vi "Sub01_Pixmap.vi"(8 "error in (no error)":errorcluster, 11 "Image Path":path) -> (0 "error out":errorcluster, 2 "Array":u32[](array[numeric]), 3 "Image Disp":picture)   [LabVIEW 2019]
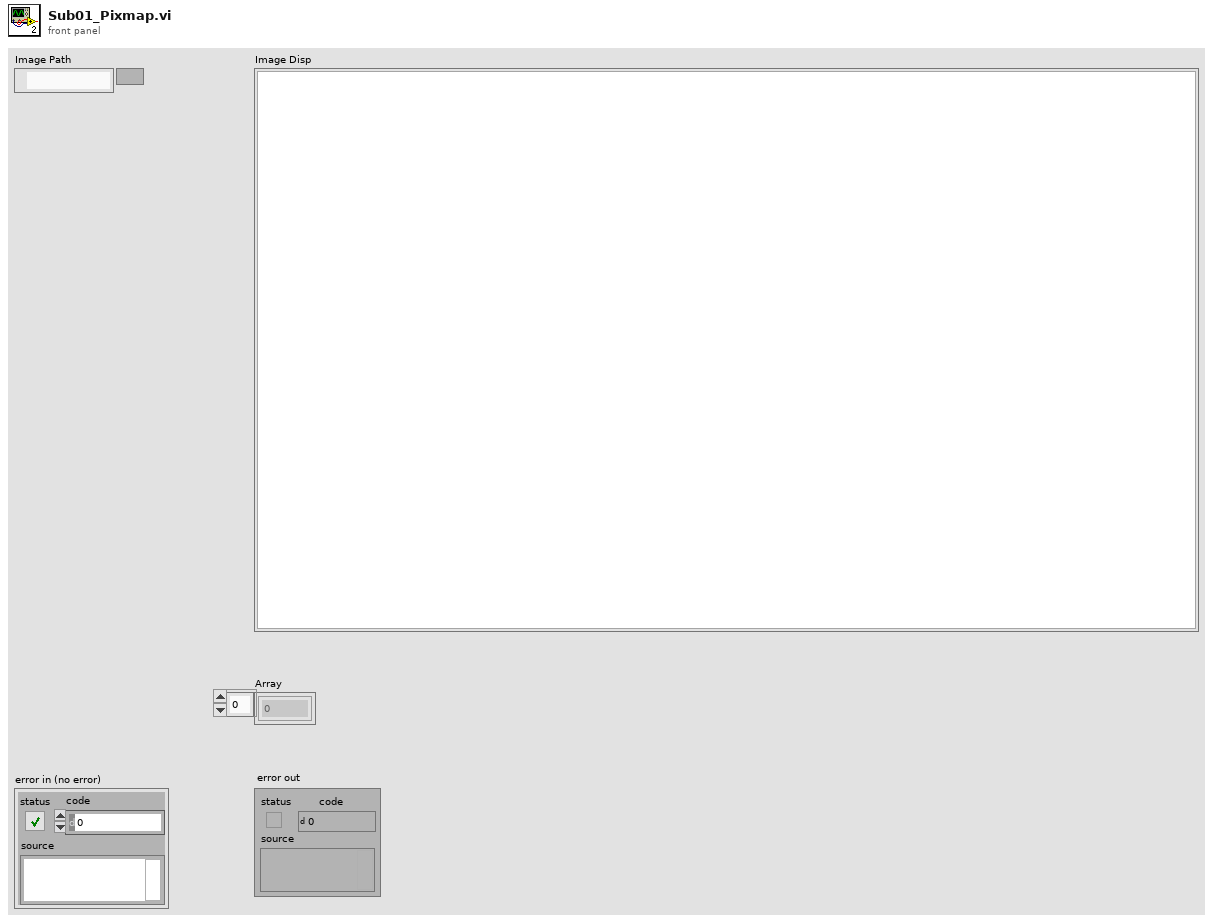
[diagram p1: front panel]
types:
  T1 = typedef "imagedata.ctl" = cluster{"image type":i32, "image depth":i32, "image":u8[], "mask":u8[], "colors":u32[], "Rectangle":cluster{"left":i16, "top":i16, "right":i16, "bottom":i16}}
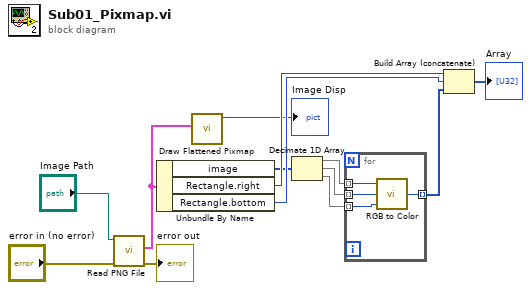
[diagram p0: block diagram]
diagram:
  n1 = call <vilib>:"Read PNG File.vi"("error in (no error)"="error in (no error)", "path to PNG file"="Image Path") -> ("error out"=→"error out":errorcluster, "image data"=w10:T1)  [unwired: 7 in, 1 out]
  n2 = Unbundle By Name(w10) -> ("image"=w5:u8[], "Rectangle.right"=w12:i16, "Rectangle.bottom"=w13:i16)
  n3 = call <vilib>:"Draw Flattened Pixmap.vi"("image data"=w10) -> ("new picture"=→"Image Disp":picture)  [unwired: 8 in]
  n4 = Decimate 1D Array(w5) -> (w4:u8[], w3:u8[], w2:u8[])
  n5 = for {
    tunnel: w4 -> [w17] mode=indexing
    tunnel: w3 -> [w16] mode=indexing
    tunnel: w2 -> [w14] mode=indexing
    tunnel: [w15] -> w1 mode=indexing
    n6 = call <vilib>:"RGB to Color.vi"("B"=w14, "G"=w16, "R"=w17) -> ("Color"=w15:u32)
  }
  n7 = Build Array (concatenate)(w12, w13, w1) -> (→"Array":u32[])
